vi "SPC_save_data_to_sdtfile.vi"(4 "Data":u16[](array[numeric]), 5 "Storing Path":path, 7 "SDT File Name":string, 8 "Error In":errorcluster, 10 "Module No":i16 min=0 max=7 step=1, 11 "DLL Path":path) -> (0 "Error Out":errorcluster, 1 "Stored to":string, 2 "Module No":i16, 3 "DLL Path":path)   [LabVIEW 2023]
doc: "This procedure saves measurement data from the buffer 'data_buf' into the 'sdt_file' file in the .sdt format using current parameters of the SPC module 'mod_no'.\n<b>The assumption is done, that before using this function user made a measurement, read the results from SPC memory and that no DLL parameters were changed in between. </b>\nBecause during the measurements always whole page(s) is affected, the best choice to read results is SPC_read_data_page function.\nThe created .sdt file can then be loaded into the SPC standard measurement software. \nIt contains a file header, an INFO section, measurement description block(s) and data set(s). It does not contain SETUP section, therefore Display, Trace, Window, Print settings will not change when the file will be loaded to SPC software.\n( for .sdt format details see SPC hardware manual and spc_minfo.h file) \nOne measurement description block and data set is created per one module (measurement description block fields are created from current 'mod_no' module's parameters).\nIn case of multi-module configuration - if 'mod_no' = -1 (all used modules), measurement description blocks and data sets are created for all modules of the same type which are 'in_use' \n( call SPC_get_module_info to know which modules are 'in_use', SPC_set_mode to change used modules configuration)\nThe 'data_buf' buffer should contain measurement data which were read earlier from SPC memory using one of memory transfer functions (SPC_read_data_page function is recommended).\nWhen 'mod_no' = -1 ( all used modules), the buffer should contain the data of all used modules in contiguous way (one after another - after last byte of 1st module's data the first byte of 2nd module should appear).\nPlease make sure that the buffer is allocated with minimum 'bytes_no' bytes, otherwise it can cause a crash.\nThe procedure checks at the beginning whether 'bytes_no' parameter fits to the current memory configuration ( use SPC_configure_memory with parameter 'adc_resolution' = -1 to get it).\n'bytes_no' must be equal to 2 * page_size * no_of_pages * no_of_modules, where\n page_size = blocks_per_frame * frames_per_page * block_length, \n no_of_pages = always 1, \n except 'Continuos Flow' mode ( for modules SPC6x0/13x/15x/160\n with mode = Normal and with sequencer enabled), \n where no_of_pages = maxpage,\n no_of_modules = 1, when 'mod_no'parameter >= 0,\n = number of active modules, when 'mod_no'parameter = -1\nDifferent measurement modes are used in .sdt file depending on the module type and current DLL parameters :\n - mode SINGLE : all module types, when DLL parameter MODE = NORMAL \n and sequencer is disabled\n - mode 'Continuos Flow' : SPC-6x0 & SPC-13x/15x/160 module types, when DLL \n parameter MODE = NORMAL and sequencer is enabled\n - mode 'Scan Sync In' : SPC-7x0/830/140/930/15x/160 module types, when \n DLL parameter MODE = SCAN_IN and sequencer is enabled\n - mode 'Scan Sync Out' : SPC-7x0/830/140/930/15x/160 module types, when \n DLL parameter MODE = SCAN_OUT and sequencer is enabled\n - mode 'Scan XY Out' : SPC-7x0 module type, when DLL parameter MODE = \n ROUT_OUT and sequencer is enabled\n - mode 'Camera' : SPC-930 module type, when DLL parameter MODE = \n CAMERA\nOther combinations of MODE value and module type are not supported and will return error. \n<b>Especially the procedure does not create the file ( returns error) when DLL parameter MODE is set to one of FIFO modes ( for modules SPC-6x0/830/13x/140/930/15x/160).</b>\nCurrently B&H is working on an extension of this procedure to also cover the FIFO modes. Until than please use the pure LabVIEW VI \\Data\\SDT Files\\SDT_WriteFile.vi in these cases.\n\ninfo@becker-hickl.com"
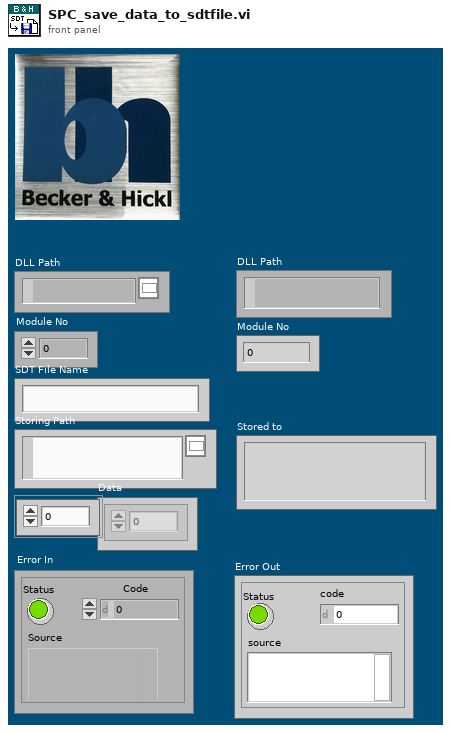
[diagram p1: front panel]
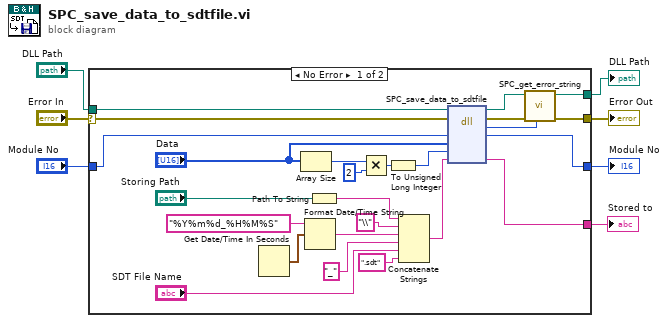
[diagram p0: block diagram]
diagram:
  n1 = case shown="No Error" "Error In" {
    selector: "Error In" -> [w12 w35]
    tunnel: [w30 w35] -> w6
    tunnel: [w26 w34] -> w5
    tunnel: "DLL Path" -> [w32 w34]
    tunnel: [w29 w33] -> w3
    tunnel: "Module No" -> [w28 w33]
    tunnel: [w13 _] -> w1
    frame No Error {
      n2 = Get Date/Time In Seconds() -> (seconds since 1Jan1904=w24:timestamp)
      n3 = Array Size(array="Data") -> (size(s)=w17:i32)
      n4 = Format Date/Time String(time format string (%c)="%Y%m%d_%H%M%S", seconds (now)=w24) -> (date/time string=w23:string)  [unwired: 1 in]
      n5 = Path To String(path="Storing Path") -> (string=w10:string)
      n6 = Multiply(x=w17, y=2) -> (x*y=w16:i32)
      n7 = To Unsigned Long Integer(number=w16) -> (unsigned 32bit integer=w8:u32)
      n8 = Concatenate Strings(w10, "\\" ("string"), w23, "_", "SDT File Name", ".sdt") -> (w9:string)
      n9 = dll-call lib="C:/Program Files (x86)/BH/SPCM/DLL/spcm64.dll" fn="SPC_save_data_to_sdtfile"(path in=w32, error in=w12, "mod_no"=w28, "data_buf"="Data", "bytes_no"=w8, "sdt_file"=w9) -> (path out=w27:path, error out=w31:errorcluster, "return type"=w25:i16, "mod_no"=w29:i16, "sdt_file"=w13:string)  [unwired: 3 in]
      n10 = call "SPC_get_error_string.vi"("ErrorID"=w25, "Error In"=w31, "DLL Path"=w27) -> ("Error Out"=w30:errorcluster, "DLL Path"=w26:path)  [unwired: 6 in, 1 out]
    }
    frame Error {
    }
  }
  "DLL Path" <- w5
  "Error Out" <- w6
  "Module No" <- w3
  "Stored to" <- w1
